vi "TRITON_RI_OPEN.vi"(2 "error in (no error)":errorcluster, 4 "Connection Details (in)":T1={"Mode"=enum."Immediate", "Bytes to Read"=5000, "IP Address"="172.25.187.107", "Remote Port"=33576, "Timeout"=10000, "connection ID"=refnum}) -> (0 "error out":errorcluster, 1 "Connection Details (out)":T1={"Mode"=enum."Immediate", "Bytes to Read"=5000, "IP Address"="172.25.187.107", "Remote Port"=33576, "Timeout"=10000, "connection ID"=refnum})   [LabVIEW 2019]
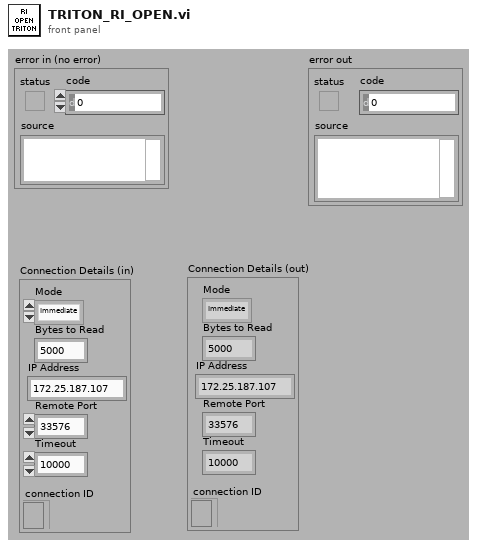
[diagram p1: front panel]
types:
  T1 = cluster{"Mode":enum16{"Standard", "Buffered", "CRLF", "Immediate"}, "Bytes to Read":i32, "IP Address":string, "Remote Port":i32, "Timeout":i32, "connection ID":refnum<k5>}
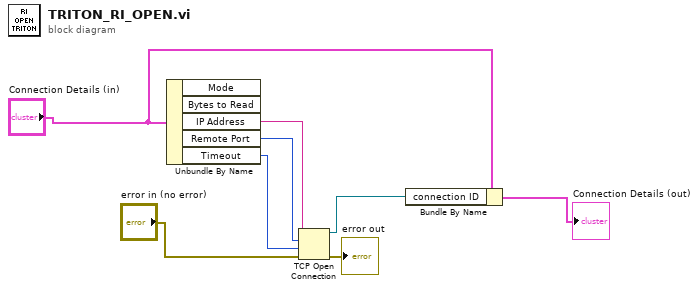
[diagram p0: block diagram]
diagram:
  n1 = Unbundle By Name("Connection Details (in)") -> ("IP Address"=w6:string, "Remote Port"=w5:i32, "Timeout"=w4:i32)  [unwired: 2 out]
  n2 = TCP Open Connection(address=w6, remote port or service name=w5, timeout ms (60000)=w4, error in (no error)="error in (no error)") -> (connection ID=w2:refnum<k5>, error out=→"error out":errorcluster)  [unwired: 1 in]
  n3 = Bundle By Name(cluster="Connection Details (in)", "connection ID"=w2) -> (→"Connection Details (out)":T1)
